vi "Read Message.vi"(4 "error in (no error)":errorcluster, 5 "timeout in ms (-1)":i32, 7 "QMH in":refnum<queue>) -> (0 "error out":errorcluster, 1 "timed out?":bool, 2 "Message":variant, 3 "Event":string)   [LabVIEW 2020, in "QHM.lvlib"]
uses:
  QHM.lvlib
  Type Defs/QMH Cluster.ctl
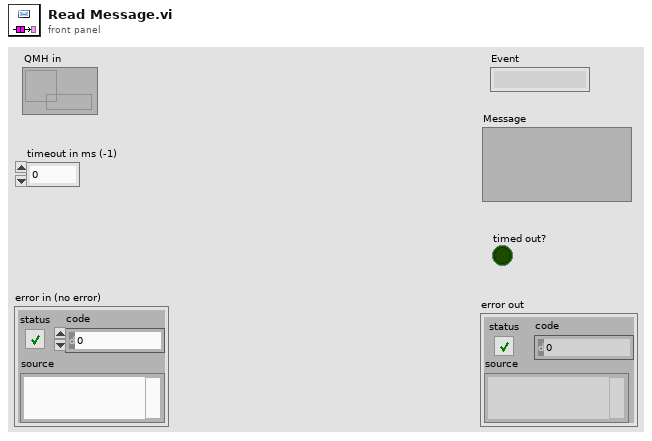
[diagram p1: front panel]
types:
  T1 = typedef "QHM.lvlib/QMH Cluster.ctl" = cluster{"Event":string, "Message":variant}
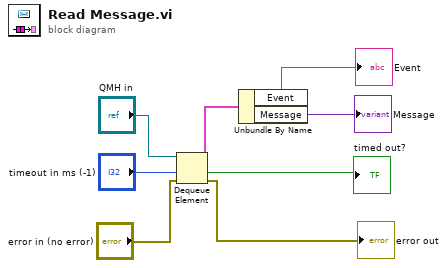
[diagram p0: block diagram]
diagram:
  n1 = Dequeue Element(queue="QMH in", timeout in ms (-1)="timeout in ms (-1)", error in (no error)="error in (no error)") -> (element=w8:T1, timed out?=→"timed out?":bool, error out=→"error out":errorcluster)  [unwired: 1 out]
  n2 = Unbundle By Name(w8) -> ("Event"=→"Event":string, "Message"=→"Message":variant)
